vi "Hatch.vi"(10 "Polys":T4[](array[typedef]), 11 "Hatch":T4) -> (3 "Path":T2)   [LabVIEW 2014]
uses:
  TypeDefs/Poly2DwSlope.ctl
  TypeDefs/Point2DwSlope.ctl
  TypeDefs/Line2D.ctl
panel:
  out "XY Graph":T3(graph)
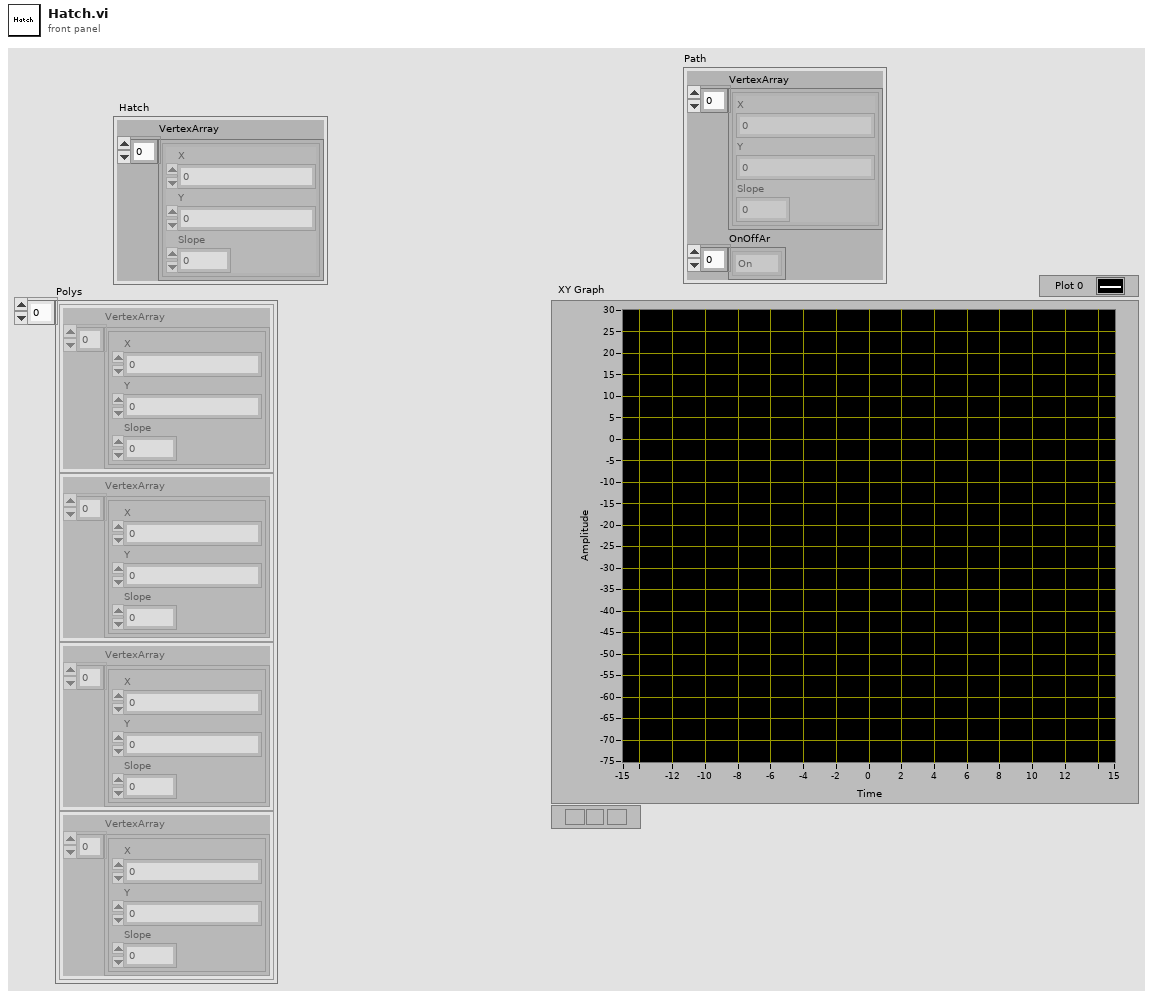
[diagram p1: front panel]
types:
  T1 = typedef "Point2DwSlope.ctl" = cluster{"X":sgl, "Y":sgl, "Slope":dbl}
  T2 = cluster{"VertexArray":T1[], "OnOffAr":enum16{"On", "Off"}[]}
  T3 = cluster{"VertexArray":cluster{"X":sgl, "Y":sgl, "Slope":dbl}[]}[]
  T4 = typedef "Poly2DwSlope.ctl" = cluster{"VertexArray":T1[]}
  T5 = typedef "Line2D.ctl" = cluster{"Vertex1":T1, "Vertex2":T1, "Slope":dbl}
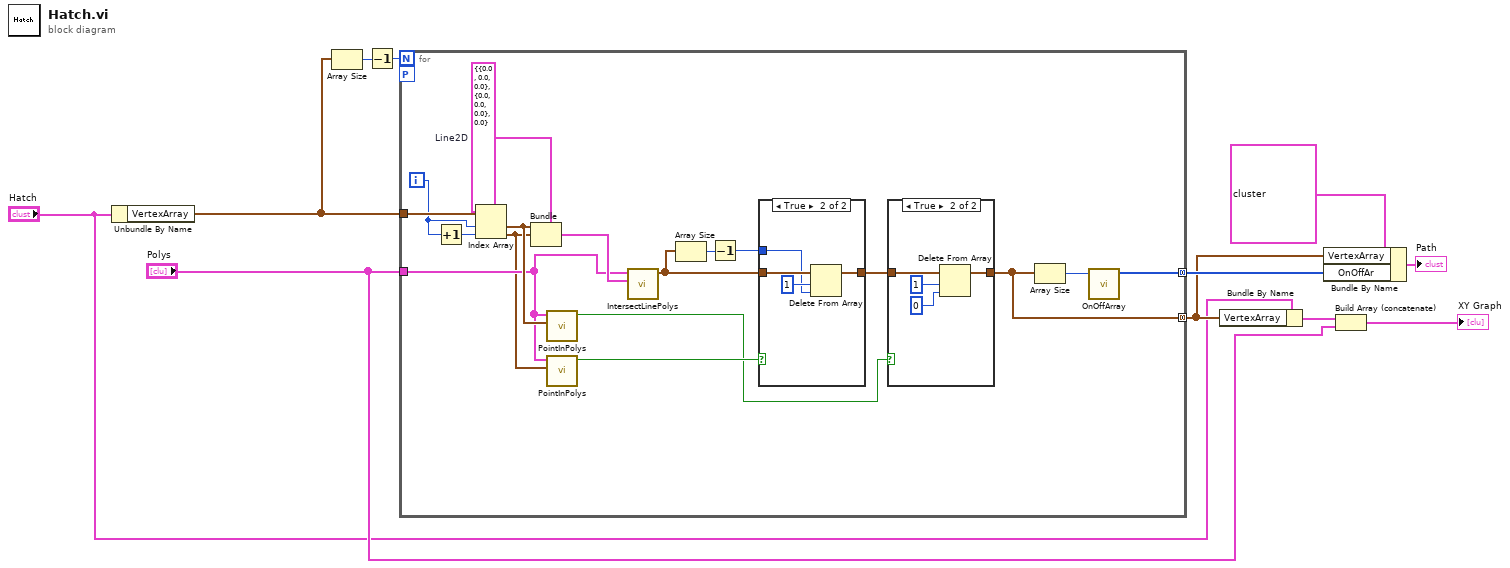
[diagram p0: block diagram]
diagram:
  n1 = Unbundle By Name("Hatch") -> ("VertexArray"=w1:T1[])
  n2 = Array Size(array=w1) -> (size(s)=w11:i32)
  n3 = Decrement(x=w11) -> (x-1=w10:i32)
  n4 = for {
    N: w10 -> [_]
    tunnel: w1 -> [w28]
    tunnel: "Polys" -> [w23]
    tunnel: [w14] -> w5 mode=concatenating
    tunnel: [w13] -> w4 mode=concatenating
    workers-P: _ -> [_]
    i -> [w26]
    w12 = T5 {"Vertex1"={"X"=0.0, "Y"=0.0, "Slope"=0.0}, "Vertex2"={"X"=0.0, "Y"=0.0, "Slope"=0.0}, "Slope"=0.0}  # Line2D
    n5 = Increment(x=w26) -> (x+1=w27:i32)
    n6 = Index Array(array=w28, index #1=w26, index #2=w27) -> (element #1=w25:T1, element #2=w22:T1)
    n7 = Bundle(cluster=w12, "Vertex1"=w25, "Vertex2"=w22) -> (w24:T5)  [unwired: 1 in]
    n8 = call "PointInPolys.vi"("Point2D"=w25, "Polys"=w23) -> ("Outside"=w16:bool)  [unwired: 9 in]
    n9 = call "PointInPolys.vi"("Point2D"=w22, "Polys"=w23) -> ("Outside"=w20:bool)  [unwired: 9 in]
    n10 = call "IntersectLinePolys.vi"("Line2D"=w24, "Polys"=w23) -> ("Intersections"=w19:T1[])  [unwired: 9 in]
    n11 = Array Size(array=w19) -> (size(s)=w21:i32)
    n12 = Decrement(x=w21) -> (x-1=w18:i32)
    n13 = case shown="True" w20 {
      tunnel: w19 -> [w34 w38]
      tunnel: w18 -> [_ w36]
      tunnel: [w34 w35] -> w17
      frame False {
      }
      frame True {
        n14 = Delete From Array(array=w38, length=1, index=w36) -> (array with subset deleted=w35:T1[])  [unwired: 1 out]
      }
    }
    n15 = case shown="True" w16 {
      tunnel: w17 -> [w29 w33]
      tunnel: [w29 w31] -> w13
      frame False {
      }
      frame True {
        n16 = Delete From Array(array=w33, length=1, index=0) -> (array with subset deleted=w31:T1[])  [unwired: 1 out]
      }
    }
    n17 = Array Size(array=w13) -> (size(s)=w15:i32)
    n18 = call "OnOffArray.vi"("Size"=w15) -> ("OnOffAr"=w14:enum16{"On", "Off"}[])  [unwired: 10 in]
  }
  n19 = Bundle By Name(cluster="Hatch", "VertexArray"=w4) -> (w9:T4)
  n20 = Bundle By Name(cluster=T2 data[14728B] ("Poly2D"), "VertexArray"=w4, "OnOffAr"=w5) -> (→"Path":T2)
  n21 = Build Array (concatenate)(w9, "Polys") -> (→"XY Graph":T4[])
